vi "模拟138译码器性能.vi"() -> ()   [LabVIEW 2012, in "触发器.lvlib"]
panel:
  out "Y7":bool
  out "Y6":bool
  out "Y5":bool
  out "Y4":bool
  out "Y3":bool
  out "Y2":bool
  out "Y1":bool
  out "Y0":bool
  in  "A2":bool
  in  "A1":bool
  in  "A0":bool
  in  "S3":bool
  in  "S2":bool
  in  "S1":bool
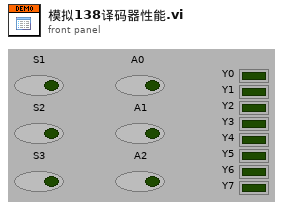
[diagram p1: front panel]
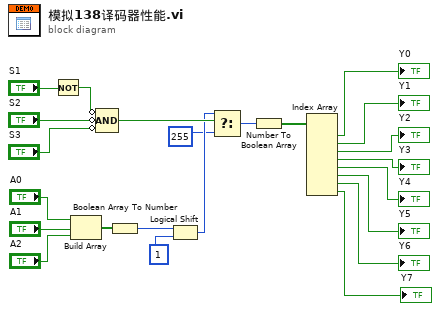
[diagram p0: block diagram]
diagram:
  n1 = Not(x="S1") -> (.not. x?=w22:bool)
  n2 = Build Array("A0", "A1", "A2") -> (w16:bool[])
  n3 = Compound Arithmetic op=AND(invert w22, invert "S2", invert "S3") -> (w15:bool)
  n4 = Boolean Array To Number(Boolean array=w16) -> (number=w14:u32)
  n5 = Logical Shift(y=w14, x=u8 1) -> (x << y=w2:u8)
  n6 = Select(t=w2, s=w15, f=u8 255) -> (s? t:f=w12:u8)
  n7 = Number To Boolean Array(number=w12) -> (Boolean array=w11:bool[])
  n8 = Index Array(array=w11) -> (element #1=→"Y0":bool, element #2=→"Y1":bool, element #3=→"Y2":bool, element #4=→"Y3":bool, element #5=→"Y4":bool, element #6=→"Y5":bool, element #7=→"Y6":bool, element #8=→"Y7":bool)  [unwired: 8 in]
